vi "Set OVP Limit.vi"(8 "error in":errorcluster, 11 "69X_79X in":refnum<class "6972A.lvclass">) -> (0 "error out":errorcluster, 3 "69X_79X out":refnum<class "6972A.lvclass">)   [LabVIEW 2019, in "6972A.lvlib" / "6972A.lvclass"]
uses:
  Library/6972A.lvclass
  C:/Users/Public/Documents/Development/builds/Instruments/PowerSupply.lvlibp/Library/PowerSupply.lvclass
  Library/6972A.lvclass/6972A.ctl
  <vilib>/Utility/error.llb/Error Cluster From Error Code.vi
  <vilib>/ErrorRing/Error Ring.xnode
  <instrlib>/Agilent N6900 N7900 Series/Agilent N6900 N7900 Series.lvlib
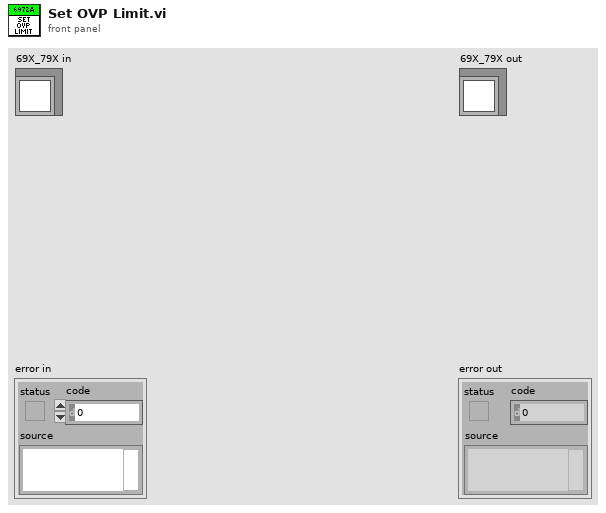
[diagram p1: front panel]
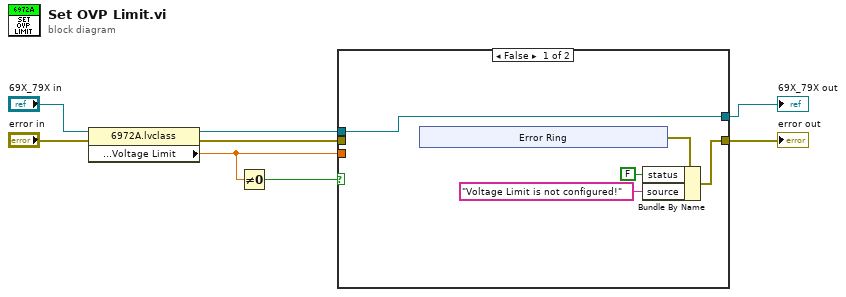
[diagram p0: block diagram]
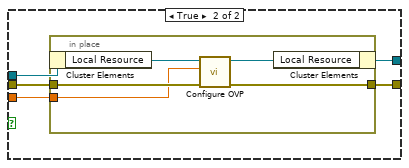
[diagram p2: hidden frame]
diagram:
  n1 = property class="6972A.lvclass"(reference="69X_79X in", error in="error in") -> (reference out=w7:refnum<class "6972A.lvclass">, error out=w5:errorcluster, "Accessors:Setting:Protection:Voltage Limit"=w2:dbl)
  n2 = Not Equal To 0?(x=w2) -> (x != 0?=w1:bool)
  n3 = case shown="False" w1 {
    tunnel: w7 -> [w13 w22]
    tunnel: [w13 w21] -> w6
    tunnel: w5 -> [_ w20]
    tunnel: [w12 w19] -> w3
    tunnel: w2 -> [_ w18]
    frame False {
      n4 = xnode "Error Ring"() -> ("error out"=w10:errorcluster)
      n5 = Bundle By Name(cluster=w10, "status"=FALSE, "source"="Voltage Limit is not configured!") -> (w12:errorcluster)
    }
    frame True {
      n6 = in-place {
        in-place-border: w20 -> [w25]
        in-place-border: w18 -> [w24]
        in-place-border: [w23] -> w19
        n7 = in-place-cluster #1(w22) -> ("Local Resource"=w27:refnum<visa-resource-name>)
        n8 = call <instrlib>:"Configure OVP.vi"("error in (no error)"=w25, "OVP Protection (48V)"=w24, "VISA resource name"=w27) -> ("error out"=w23:errorcluster, "VISA resource name out"=w26:refnum<visa-resource-name>)  [unwired: 7 in]
        n9 = in-place-cluster #1("Local Resource"=w26) -> (w21:refnum<class "6972A.lvclass">)
      }
    }
  }
  "error out" <- w3
  "69X_79X out" <- w6
